vi "Read Append Numeric.vi"(11 "StringIncrement":refnum<class "StringIncrement.lvclass">) -> (2 "Append Numeric":u32, 3 "StringIncrement out":refnum<class "StringIncrement.lvclass">)   [LabVIEW 2013, in "UniqueName.lvlib" / "StringIncrement.lvclass"]
uses:
  StringIncrement.lvclass
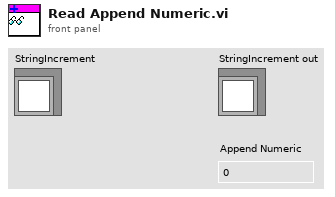
[diagram p1: front panel]
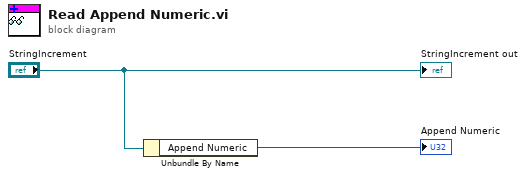
[diagram p0: block diagram]
diagram:
  n1 = Unbundle By Name("StringIncrement") -> ("Append Numeric"=→"Append Numeric":u32)
  "StringIncrement out" <- "StringIncrement"
